vi "niWLAN - OPPO - 80211abgnIQMeasurements.vi"(0 "niwlan analysis session":T5, 2 "Measurement Type":T3(ring), 3 "PL":T2, 7 "TV Parameters(DataType)":T4 {"Standard" items=["80211A/G/J/P OFDM", "80211B/G DSSS", "80211G DSSSOFDM", "80211N MIMOOFDM", "80211AC MIMOOFDM"]; "OFDM Data Rate (Mbps)" items=["6", "9", "12", "18", "24", "36", "48", "54"]; "80211n PLCP Frame Format" items=["Mixed Format", "Greenfield Format"]; "FEC Coding Type" items=["BCC", "LDPC"]; "DSSS Data Rate (Mbps)" items=["1", "2", "5.5 CCK", "5.5 PBCC", "11 CCK", "11 PBCC", "22", "33"]}, 11 "error out":errorcluster) -> (4 "niWLAN session":T5, 6 "Spectrum Result":cluster{"SMM":dbl, "SMM VECTOR":dbl[]}, 8 "Mod Result":T1={"EVM"=-53.23630011850784, "RMS POWER"=-20.854257366141734, "FREQ ERR PPm"=0.0031004693085368165, "Clock ERR PPm"=1.9815491854025864}, 15 "error out":errorcluster)   [LabVIEW 2012]
uses:
  <vilib>/RF Toolkits/WLAN/analysis/controls/wlanv1 Analysis Refnum.ctl
  TV/RW/Includes/WLAN - TV - RW - INC - TV_DataType_Cluster.ctl
  TV/RW/Includes/WLAN - TV - RW - INC - Tx_IQModResult.ctl
  <resource>/objmgr/niWLANAnalysis.rc
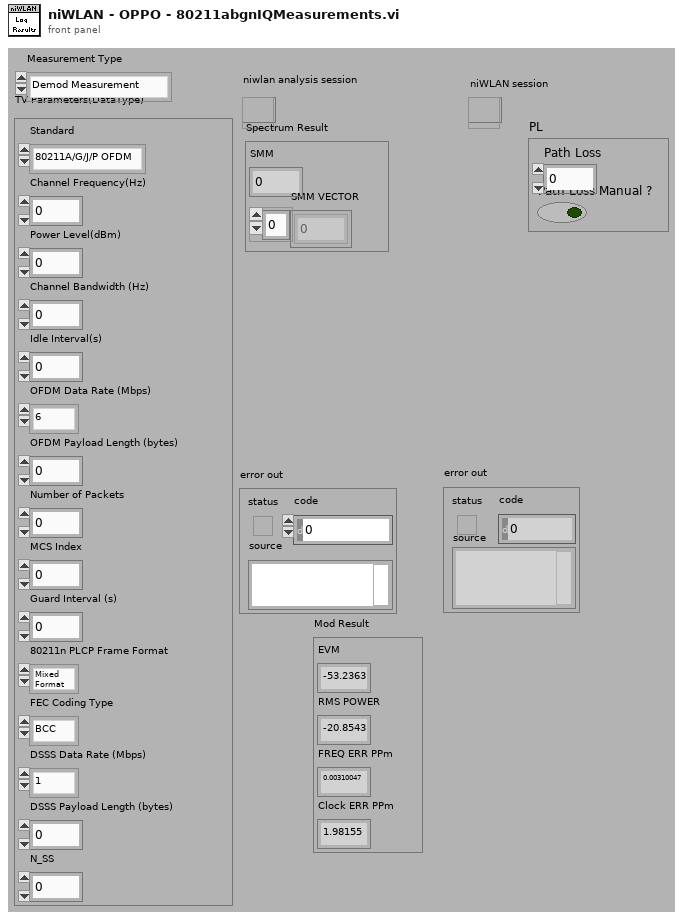
[diagram p1: front panel]
types:
  T1 = typedef "WLAN - TV - RW - INC - Tx_IQModResult.ctl" = cluster{"EVM":dbl, "RMS POWER":dbl, "FREQ ERR PPm":dbl, "Clock ERR PPm":dbl}
  T2 = cluster{"Path Loss":dbl, "Path Loss Manual ?":bool}
  T3 = enum16{"Demod Measurement", "Spectrum Measurement"}
  T4 = typedef "WLAN - TV - RW - INC - TV_DataType_Cluster.ctl" = cluster{"Standard":i32, "Channel Frequency(Hz)":dbl, "Power Level(dBm)":dbl, "Channel Bandwidth (Hz)":dbl, "Idle Interval(s)":dbl, "OFDM Data Rate (Mbps)":i32, "OFDM Payload Length (bytes)":i32, "Number of Packets":i32, "MCS Index":i32, "Guard Interval (s)":dbl, "80211n PLCP Frame Format":i32, "FEC Coding Type":i32, "DSSS Data Rate (Mbps)":i32, "DSSS Payload Length (bytes)":i32, "N_SS":i32}
  T5 = typedef "wlanv1 Analysis Refnum.ctl" = refnum<k20>
  T6 = cluster{"subcarrier indices":i32[], "relative power (dB)":dbl[]}
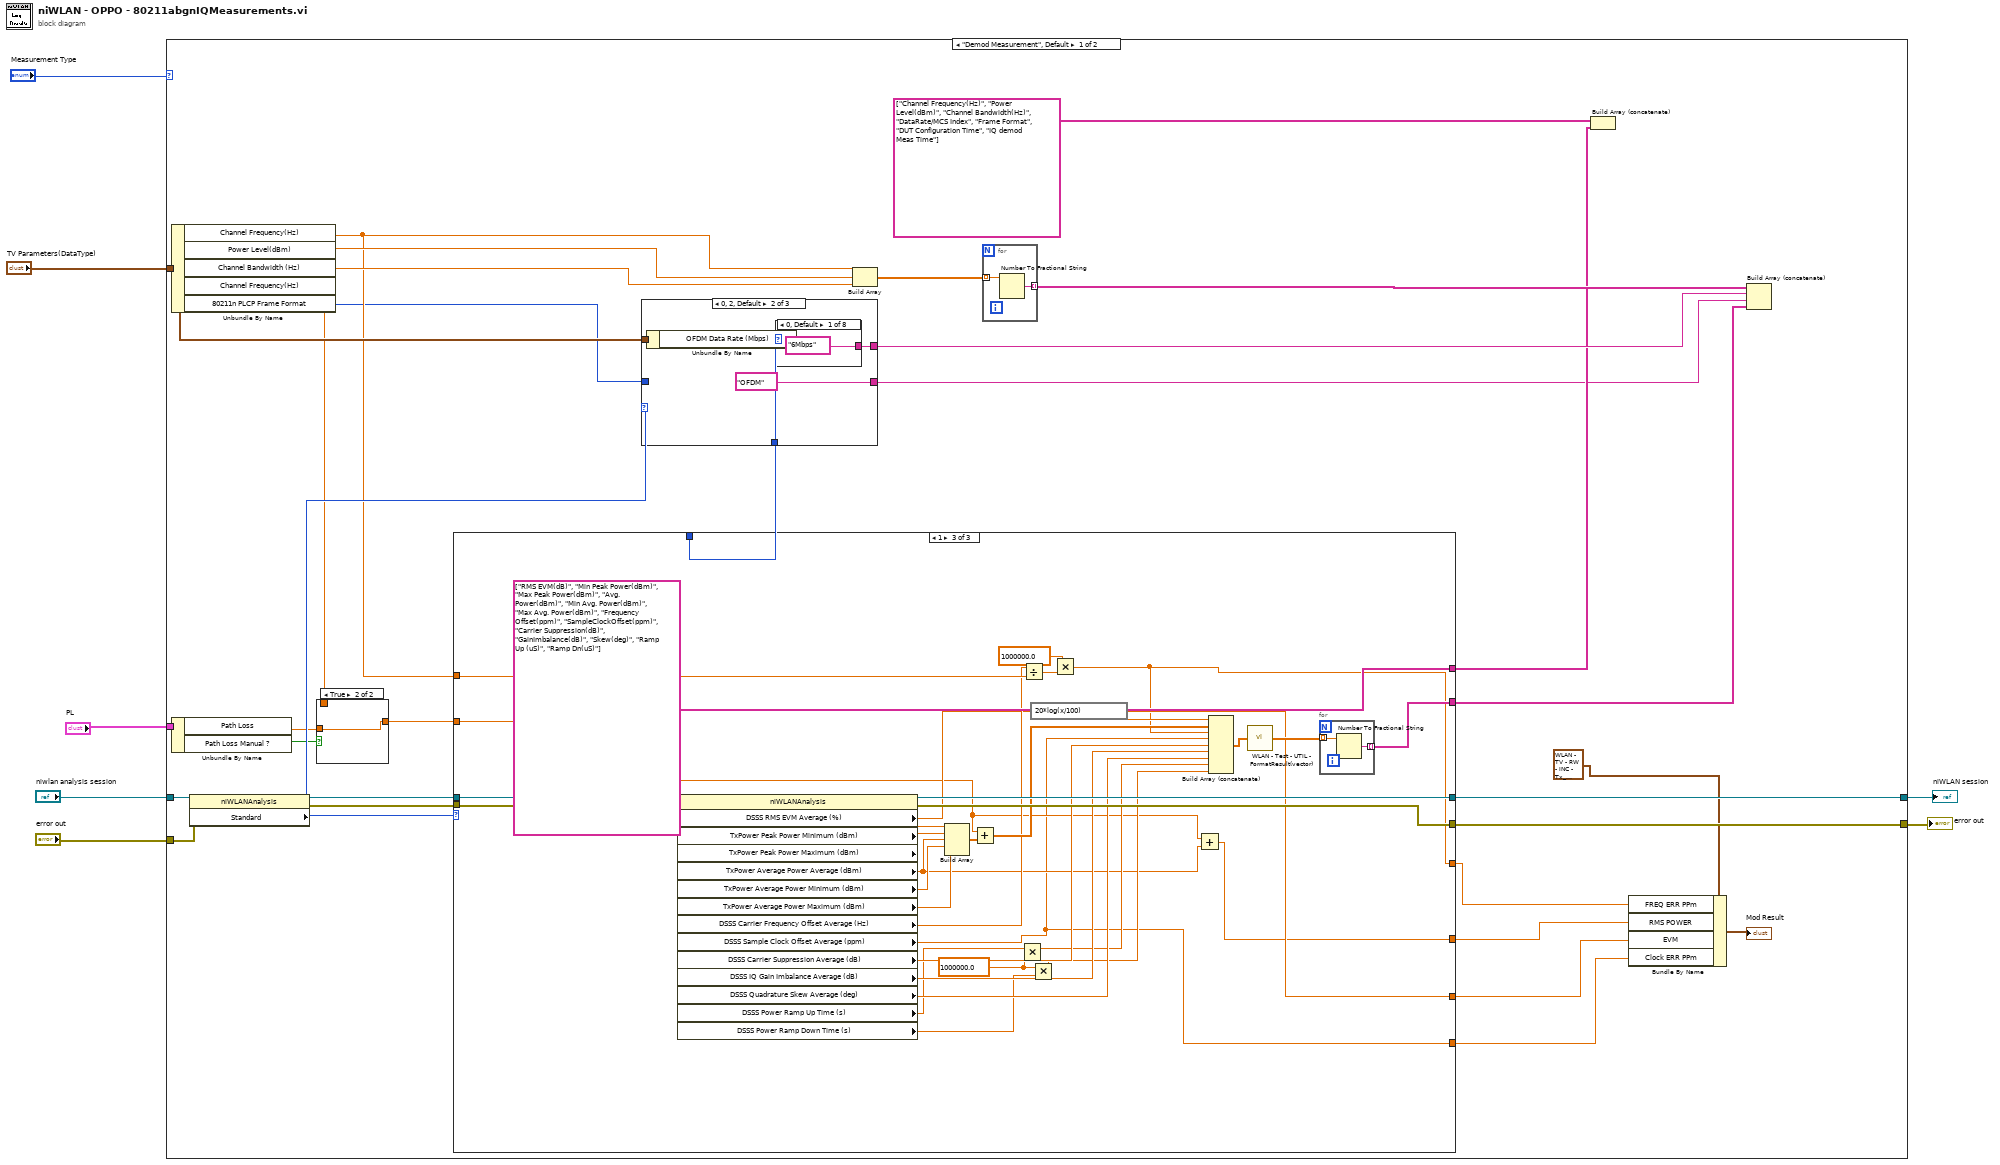
[diagram p0: block diagram]
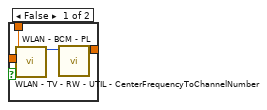
[diagram p2: hidden frame]
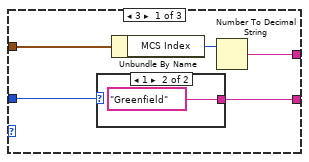
[diagram p3: hidden frame]
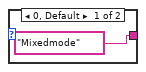
[diagram p4: hidden frame]
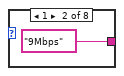
[diagram p5: hidden frame]
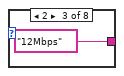
[diagram p6: hidden frame]
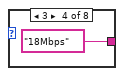
[diagram p7: hidden frame]
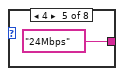
[diagram p8: hidden frame]
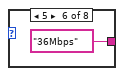
[diagram p9: hidden frame]
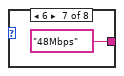
[diagram p10: hidden frame]
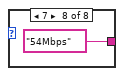
[diagram p11: hidden frame]
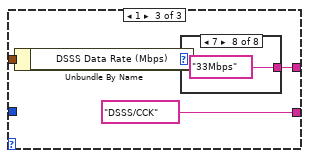
[diagram p12: hidden frame]
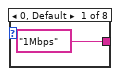
[diagram p13: hidden frame]
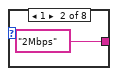
[diagram p14: hidden frame]
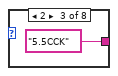
[diagram p15: hidden frame]
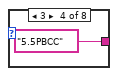
[diagram p16: hidden frame]
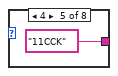
[diagram p17: hidden frame]
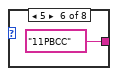
[diagram p18: hidden frame]
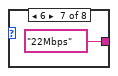
[diagram p19: hidden frame]
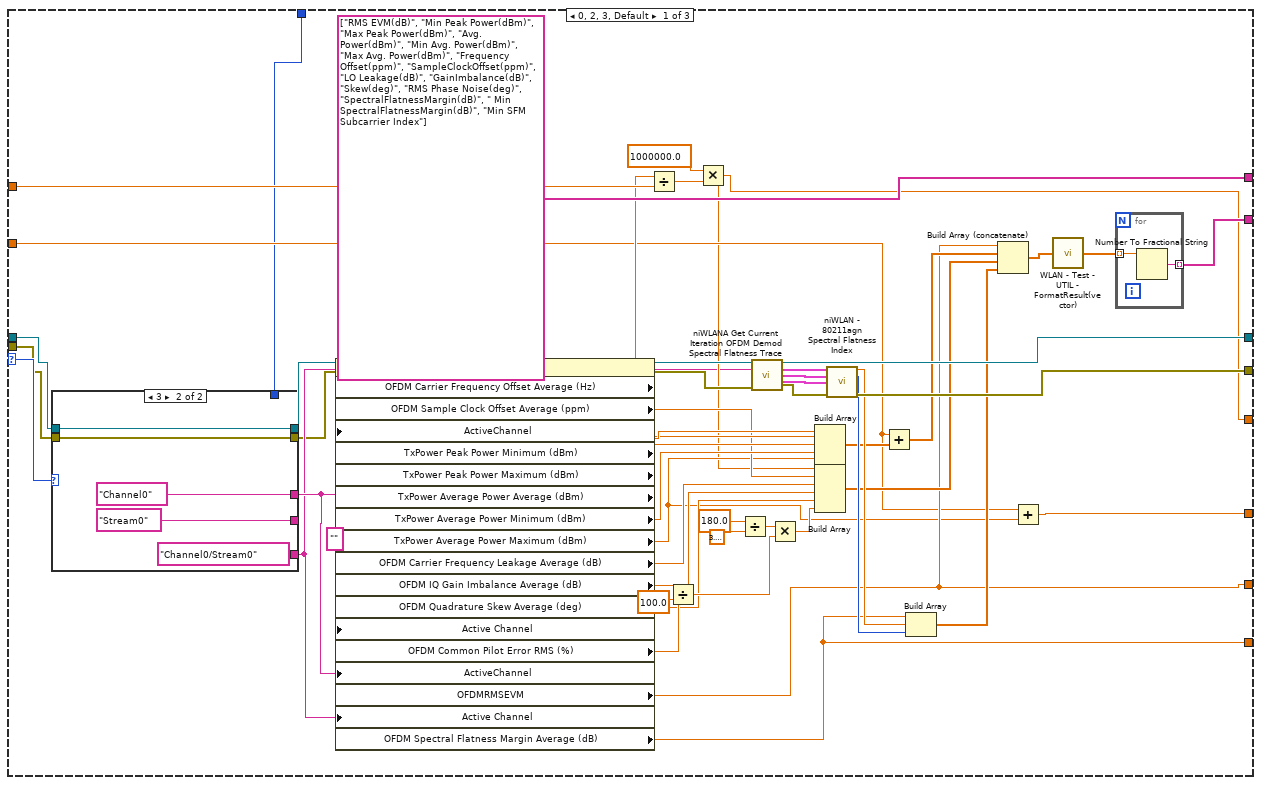
[diagram p20: hidden frame]
diagram:
  n1 = case shown="\"Demod Measurement\", Default" "Measurement Type" {
    tunnel: "niwlan analysis session" -> [w38 w264]
    tunnel: "error out" -> [w36 w265]
    tunnel: "TV Parameters(DataType)" -> [w29 w266]
    tunnel: [w24 w262] -> w4
    tunnel: [w23 w263] -> w3
    tunnel: "PL" -> [w17 _]
    frame "Demod Measurement", Default {
      n2 = Unbundle By Name(w29) -> ("Channel Frequency(Hz)"=w25:dbl, "Power Level(dBm)"=w33:dbl, "Channel Bandwidth (Hz)"=w32:dbl, "Channel Frequency(Hz)"=w20:dbl, "80211n PLCP Frame Format"=w19:i32)
      n3 = Unbundle By Name(w17) -> ("Path Loss"=w15:dbl, "Path Loss Manual ?"=w16:bool)
      n4 = property class="niWLANAnalysis"(reference=w38, error in=w36) -> (reference out=w37:T5, error out=w35:errorcluster, "Standard"=w28:i32)
      n5 = case shown="True" w16 {
        tunnel: [w41 w42] -> w21
        tunnel: w20 -> [w39 _]
        tunnel: w15 -> [_ w42]
        frame False {
          n6 = call "WLAN - TV - RW - UTIL - CenterFrequencyToChannelNumber.vi"("Center Frequency(Hz)"=w39) -> ("Coherced Channel Number"=w40:i32)  [unwired: 13 in, 1 out]
          n7 = call "WLAN - BCM - PL.vi"("Channel index"=w40) -> ("PL"=w41:dbl)  [unwired: 10 in]
        }
        frame True {
        }
      }
      n8 = case shown="1" w28 {
        selector: w28 -> [w127 _ _]
        tunnel: w35 -> [w108 w145 w222]
        tunnel: w37 -> [w77 w146 w223]
        tunnel: [w106 w170 w221] -> w24
        tunnel: [w103 w167 w220] -> w23
        tunnel: [w126 w188 w216] -> w14
        tunnel: [string[] ["RMS EVM(dB)", "Min Peak Power(dBm)", "Max Peak Power(dBm)", "Avg. Power(dBm)", "Min Avg. Power(dBm)", "Max Avg. Power(dBm)", "Frequency Offset(ppm)", "SampleClockOffset(ppm)", "LO Leakage(dB)", "GainImbalance(dB)", "Skew(deg)", "RMS Phase Noise(deg)", "SpectralFlatnessMargin(dB)", " Min SpectralFlatnessMargin(dB)", "Min SFM Subcarrier Index"] string[] ["RMS EVM(dB)", "Min Peak Power(dBm)", "Max Peak Power(dBm)", "Avg. Power(dBm)", "Min Avg. Power(dBm)", "Max Avg. Power(dBm)", "Frequency Offset(ppm)", "SampleClockOffset(ppm)", "LO Leakage(dB)", "GainImbalance(dB)", "Skew(deg)", "RMS Phase Noise(deg)", "SpectralFlatnessMargin(dB)", " Min SpectralFlatnessMargin(dB)", "Min SFM Subcarrier Index"] string[] ["RMS EVM(dB)", "Min Peak Power(dBm)", "Max Peak Power(dBm)", "Avg. Power(dBm)", "Min Avg. Power(dBm)", "Max Avg. Power(dBm)", "Frequency Offset(ppm)", "SampleClockOffset(ppm)", "Carrier Suppression(dB)", "GainImbalance(dB)", "Skew(deg)", "Ramp Up (uS)", "Ramp Dn(uS)"]] -> w26
        tunnel: w25 -> [w122 w184 w215]
        tunnel: [w78 _ _] -> w22
        tunnel: w21 -> [w83 w149 w195]
        tunnel: [w81 w147 w196] -> w12
        tunnel: [w86 w152 w197] -> w10
        tunnel: [w85 w151 w191] -> w13
        tunnel: [w82 w148 w193] -> w11
        frame 0, 2, 3, Default {
          n9 = case shown="3" w127 {
            tunnel: [w135 "Channel0/Stream0"] -> w80
            tunnel: [w135 "Stream0" ("Active Channel")] -> _
            tunnel: [w135 "Channel0" ("Active Channel")] -> w88
            tunnel: w77 -> [w134 w136]
            tunnel: w108 -> [w133 w137]
            tunnel: [w132 w137] -> w79
            tunnel: [w131 _] -> w78
            tunnel: [w130 w136] -> w76
            frame 0, 2, Default {
              w135 = "" ("Active Channel")
              n10 = property class="niWLANAnalysis"(reference=w134, error in=w133) -> (reference out=w130:T5, error out=w132:errorcluster, "Detected OFDM Data Rate (Mbps)"=w131:i32)
            }
            frame 3 {
            }
          }
          n11 = property class="niWLANAnalysis"(reference=w76, error in=w79, "ActiveChannel"=w88, "Active Channel"="", "ActiveChannel"=w88, "Active Channel"=w80) -> (reference out=w107:T5, error out=w105:errorcluster, "OFDM Carrier Frequency Offset Average (Hz)"=w87:dbl, "OFDM Sample Clock Offset Average (ppm)"=w97:dbl, "TxPower Peak Power Minimum (dBm)"=w119:dbl, "TxPower Peak Power Maximum (dBm)"=w118:dbl, "TxPower Average Power Average (dBm)"=w117:dbl, "TxPower Average Power Minimum (dBm)"=w116:dbl, "TxPower Average Power Maximum (dBm)"=w84:dbl, "OFDM Carrier Frequency Leakage Average (dB)"=w96:dbl, "OFDM IQ Gain Imbalance Average (dB)"=w95:dbl, "OFDM Quadrature Skew Average (deg)"=w94:dbl, "OFDM Common Pilot Error RMS (%)"=w109:dbl, "OFDMRMSEVM"=w86:dbl, "OFDM Spectral Flatness Margin Average (dB)"=w85:dbl)
          n12 = Divide(x=w87, y=w122) -> (x/y=w124:dbl)
          n13 = Divide(x=w109, y=100.0 ("x")) -> (x/y=w114:dbl)
          n14 = Multiply(x=1000000.0, y=w124) -> (x*y=w81:dbl)
          n15 = Divide(x=180.0, y=3.141592653589793) -> (x/y=w111:dbl)
          n16 = call <vilib>:"niWLANA Get Current Iteration OFDM Demod Spectral Flatness Trace.vi"("niwlan analysis session"=w107, "active channel"=w80, "error in"=w105) -> ("niwlan analysis session out"=w106:T5, "spectral flatness upper mask"=w102:T6, "spectral flatness trace"=w101:T6, "spectral flatness lower mask"=w100:T6, "error out"=w104:errorcluster)  [unwired: 8 in]
          n17 = Multiply(x=w111, y=w114) -> (x*y=w93:dbl)
          n18 = Build Array(w119, w118, w117, w116, w84) -> (w92:dbl[])
          n19 = Build Array(w81, w97, w96, w95, w94, w93) -> (w89:dbl[])
          n20 = call "niWLAN - 80211agn Spectral Flatness Index.vi"("spectral flatness upper mask"=w102, "spectral flatness Trace"=w101, "spectral flatness Lower mask"=w100, "error in (no error)"=w104) -> ("Least Spectral Flatness Margin"=w98:dbl, "Spectral Flatness Margin Subcarrier Index"=w99:i32, "error out"=w103:errorcluster)  [unwired: 9 in]
          n21 = Add(x=w83, y=w92) -> (x+y=w91:dbl[])
          n22 = Build Array(w85, w98, w99) -> (w90:dbl[])
          n23 = Build Array (concatenate)(w86, w91, w89, w90) -> (w121:dbl[])
          n24 = Add(x=w83, y=w84) -> (x+y=w82:dbl)
          n25 = call "WLAN - Test - UTIL - FormatResult(vector).vi"("Number"=w121) -> ("2nd order decimal"=w120:dbl[])  [unwired: 14 in]
          n26 = for {
            tunnel: [w129] -> w126 mode=indexing
            tunnel: w120 -> [w128] mode=indexing
            n27 = Number To Fractional String(number=w128) -> (F-format string=w129:string)  [unwired: 3 in]
          }
        }
        frame 4 {
          w141 = "Segment0/Channel0/Stream0" ("Active Channel")
          w142 = "Segment0/Channel0" ("Active Channel")
          n28 = property class="niWLANAnalysis"(reference=w146, error in=w145, "Active Channel"="Segment0", "ActiveChannel"=w142, "Active Channel"=w142, "ActiveChannel"=w142, "Active Channel"=w141) -> (reference out=w171:T5, error out=w169:errorcluster, "OFDM Carrier Frequency Offset Average (Hz)"=w144:dbl, "OFDM Sample Clock Offset Average (ppm)"=w161:dbl, "TxPower Peak Power Minimum (dBm)"=w181:dbl, "TxPower Peak Power Maximum (dBm)"=w180:dbl, "TxPower Average Power Average (dBm)"=w179:dbl, "TxPower Average Power Minimum (dBm)"=w178:dbl, "TxPower Average Power Maximum (dBm)"=w150:dbl, "OFDM Carrier Frequency Leakage Average (dB)"=w160:dbl, "OFDM IQ Gain Imbalance Average (dB)"=w159:dbl, "OFDM Quadrature Skew Average (deg)"=w158:dbl, "OFDM Common Pilot Error RMS (%)"=w172:dbl, "OFDMRMSEVM"=w152:dbl, "OFDM Spectral Flatness Margin Average (dB)"=w151:dbl)
          n29 = Divide(x=w144, y=w184) -> (x/y=w186:dbl)
          n30 = Divide(x=w172, y=100.0 ("x")) -> (x/y=w177:dbl)
          n31 = Multiply(x=1000000.0, y=w186) -> (x*y=w147:dbl)
          n32 = Divide(x=180.0, y=3.141592653589793) -> (x/y=w174:dbl)
          n33 = call <vilib>:"niWLANA Get Current Iteration OFDM Demod Spectral Flatness Trace.vi"("niwlan analysis session"=w171, "active channel"=w141, "error in"=w169) -> ("niwlan analysis session out"=w170:T5, "spectral flatness upper mask"=w166:T6, "spectral flatness trace"=w165:T6, "spectral flatness lower mask"=w164:T6, "error out"=w168:errorcluster)  [unwired: 8 in]
          n34 = Multiply(x=w174, y=w177) -> (x*y=w157:dbl)
          n35 = Build Array(w181, w180, w179, w178, w150) -> (w156:dbl[])
          n36 = Build Array(w147, w161, w160, w159, w158, w157) -> (w153:dbl[])
          n37 = call "niWLAN - 80211agn Spectral Flatness Index.vi"("spectral flatness upper mask"=w166, "spectral flatness Trace"=w165, "spectral flatness Lower mask"=w164, "error in (no error)"=w168) -> ("Least Spectral Flatness Margin"=w162:dbl, "Spectral Flatness Margin Subcarrier Index"=w163:i32, "error out"=w167:errorcluster)  [unwired: 9 in]
          n38 = Add(x=w149, y=w156) -> (x+y=w155:dbl[])
          n39 = Build Array(w151, w162, w163) -> (w154:dbl[])
          n40 = Build Array (concatenate)(w152, w155, w153, w154) -> (w183:dbl[])
          n41 = Add(x=w149, y=w150) -> (x+y=w148:dbl)
          n42 = call "WLAN - Test - UTIL - FormatResult(vector).vi"("Number"=w183) -> ("2nd order decimal"=w182:dbl[])  [unwired: 14 in]
          n43 = for {
            tunnel: [w190] -> w188 mode=indexing
            tunnel: w182 -> [w189] mode=indexing
            n44 = Number To Fractional String(number=w189) -> (F-format string=w190:string)  [unwired: 3 in]
          }
        }
        frame 1 {
          w200 = 1000000.0 ("x")
          n45 = property class="niWLANAnalysis"(reference=w223, error in=w222) -> (reference out=w221:T5, error out=w220:errorcluster, "DSSS RMS EVM Average (%)"=w198:dbl, "TxPower Peak Power Minimum (dBm)"=w209:dbl, "TxPower Peak Power Maximum (dBm)"=w208:dbl, "TxPower Average Power Average (dBm)"=w192:dbl, "TxPower Average Power Minimum (dBm)"=w207:dbl, "TxPower Average Power Maximum (dBm)"=w194:dbl, "DSSS Carrier Frequency Offset Average (Hz)"=w199:dbl, "DSSS Sample Clock Offset Average (ppm)"=w191:dbl, "DSSS Carrier Suppression Average (dB)"=w219:dbl, "DSSS IQ Gain Imbalance Average (dB)"=w218:dbl, "DSSS Quadrature Skew Average (deg)"=w217:dbl, "DSSS Power Ramp Up Time (s)"=w204:dbl, "DSSS Power Ramp Down Time (s)"=w203:dbl)
          n46 = Build Array(w209, w208, w192, w207, w194) -> (w206:dbl[])
          n47 = Add(x=w195, y=w206) -> (x+y=w205:dbl[])
          n48 = Multiply(x=w204, y=w200) -> (x*y=w202:dbl)
          n49 = Divide(x=w199, y=w215) -> (x/y=w214:dbl)
          n50 = expression code="20*log(x/100)"(w198) -> (w197:dbl)
          n51 = Multiply(x=w200, y=w203) -> (x*y=w201:dbl)
          n52 = Multiply(x=1000000.0, y=w214) -> (x*y=w196:dbl)
          n53 = Add(x=w195, y=w192) -> (x+y=w193:dbl)
          n54 = Build Array (concatenate)(w197, w205, w196, w191, w219, w218, w217, w202, w201) -> (w211:dbl[])
          n55 = call "WLAN - Test - UTIL - FormatResult(vector).vi"("Number"=w211) -> ("2nd order decimal"=w210:dbl[])  [unwired: 14 in]
          n56 = for {
            tunnel: [w225] -> w216 mode=indexing
            tunnel: w210 -> [w224] mode=indexing
            n57 = Number To Fractional String(number=w224) -> (F-format string=w225:string)  [unwired: 3 in]
          }
        }
      }
      n58 = case shown="0, 2, Default" w28 {
        tunnel: [w47 "OFDM" ("active channel") "DSSS/CCK" ("active channel")] -> w18
        tunnel: w29 -> [w46 w52 w64]
        tunnel: [w44 w51 w62] -> w30
        tunnel: w22 -> [_ w50 _]
        tunnel: w19 -> [w43 _ _]
        frame 3 {
          n59 = case shown="1" w43 {
            tunnel: ["Mixedmode" ("active channel") "Greenfield" ("active channel")] -> w47
            frame 0, Default {
            }
            frame 1 {
            }
          }
          n60 = Unbundle By Name(w46) -> ("MCS Index"=w45:i32)
          n61 = Number To Decimal String(number=w45) -> (decimal integer string=w44:string)  [unwired: 1 in]
        }
        frame 0, 2, Default {
          n62 = Unbundle By Name(w52) -> ()  [unwired: 1 out]
          n63 = case shown="0, Default" w50 {
            tunnel: ["6Mbps" ("active channel") "9Mbps" ("active channel") "12Mbps" ("active channel") "18Mbps" ("active channel") "24Mbps" ("active channel") "36Mbps" ("active channel") "48Mbps" ("active channel") "54Mbps" ("active channel")] -> w51
            frame 0, Default {
            }
            frame 1 {
            }
            frame 2 {
            }
            frame 3 {
            }
            frame 4 {
            }
            frame 5 {
            }
            frame 6 {
            }
            frame 7 {
            }
          }
        }
        frame 1 {
          n64 = Unbundle By Name(w64) -> ("DSSS Data Rate (Mbps)"=w63:i32)
          n65 = case shown="7" w63 {
            tunnel: ["1Mbps" ("active channel") "2Mbps" ("active channel") "5.5CCK" ("active channel") "5.5PBCC" ("active channel") "11CCK" ("active channel") "11PBCC" ("active channel") "22Mbps" ("active channel") "33Mbps" ("active channel")] -> w62
            frame 0, Default {
            }
            frame 1 {
            }
            frame 2 {
            }
            frame 3 {
            }
            frame 4 {
            }
            frame 5 {
            }
            frame 6 {
            }
            frame 7 {
            }
          }
        }
      }
      n66 = Build Array(w25, w33, w32) -> (w34:dbl[])
      n67 = for {
        tunnel: [w75] -> w31 mode=indexing
        tunnel: w34 -> [w74] mode=indexing
        n68 = Number To Fractional String(number=w74) -> (F-format string=w75:string)  [unwired: 3 in]
      }
      n69 = Build Array (concatenate)(string[] ["Channel Frequency(Hz)", "Power Level(dBm)", "Channel Bandwidth(Hz)", "DataRate/MCS Index", "Frame Format", "DUT Configuration Time", "IQ demod Meas Time"], w26) -> ()  [unwired: 1 out]
      n70 = Bundle By Name(cluster=T1 {"EVM"=-53.23630011850784, "RMS POWER"=-20.854257366141734, "FREQ ERR PPm"=0.0031004693085368165, "Clock ERR PPm"=1.9815491854025864} ("Mod Result"), "FREQ ERR PPm"=w12, "RMS POWER"=w11, "EVM"=w10, "Clock ERR PPm"=w13) -> (→"Mod Result":T1)
      n71 = Build Array (concatenate)(w31, w30, w18, w14) -> ()  [unwired: 1 out]
    }
    frame "Spectrum Measurement" {
      n72 = property class="niWLANAnalysis"(reference=w264, error in=w265) -> (reference out=w261:T5, error out=w260:errorcluster, "Standard"=w259:i32)
      n73 = case shown="3" w259 {
        tunnel: ["Channel0" ("active channel") "Segment0/Channel0" ("active channel") "" ("active channel") "" ("active channel")] -> w235
        tunnel: w266 -> [w278 w288 w294 w308]
        tunnel: [w274 w284 w292 w306] -> w237
        tunnel: [string[] ["SMM(-33MHz  -  -30MHz) ", "SMM(dB)(-30MHz  -  -20MHz) ", "SMM(dB)(-20MHz  -  -11MHz) ", "SMM(dB)(-11MHz  -  -9MHz) ", "SMM(dB)(-9MHz  -  9MHz) ", "SMM(dB)(9MHz  -  11MHz) ", "SMM(dB)(11MHz  -  20MHz) ", "SMM(dB)(20MHz  -  30MHz) ", "SMM(dB)(30MHz  -  33MHz) "] string[] ["SMM(-33MHz  -  -30MHz) ", "SMM(dB)(-30MHz  -  -20MHz) ", "SMM(dB)(-20MHz  -  -11MHz) ", "SMM(dB)(-11MHz  -  -9MHz) ", "SMM(dB)(-9MHz  -  9MHz) ", "SMM(dB)(9MHz  -  11MHz) ", "SMM(dB)(11MHz  -  20MHz) ", "SMM(dB)(20MHz  -  30MHz) ", "SMM(dB)(30MHz  -  33MHz) "] string[] ["SMM(-33MHz  -  -30MHz) ", "SMM(dB)(-30MHz  -  -20MHz) ", "SMM(dB)(-20MHz  -  -11MHz) ", "SMM(dB)(-11MHz  -  -9MHz) ", "SMM(dB)(-9MHz  -  9MHz) ", "SMM(dB)(9MHz  -  11MHz) ", "SMM(dB)(11MHz  -  20MHz) ", "SMM(dB)(20MHz  -  30MHz) ", "SMM(dB)(30MHz  -  33MHz) "] string[] ["SMM(-33MHz  -  -22MHz) ", "SMM(-22MHz  -  -11MHz) ", "SMM(-11MHz  -  11MHz) ", "SMM(11MHz  -  22MHz) ", "SMM(22MHz  -  33MHz) "]] -> w234
        tunnel: [w272 "OFDM" ("active channel") "OFDM" ("active channel") "DSSS/CCK" ("active channel")] -> w231
        frame 3 {
          n74 = Unbundle By Name(w278) -> ("MCS Index"=w277:i32, "80211n PLCP Frame Format"=w273:i32)
          n75 = case shown="0, Default" w273 {
            tunnel: ["Mixedmode" ("active channel") "Greenfield" ("active channel")] -> w272
            frame 0, Default {
            }
            frame 1 {
            }
          }
          n76 = Number To Decimal String(number=w277) -> (decimal integer string=w275:string)  [unwired: 1 in]
          n77 = Concatenate Strings("MCS " ("string"), w275) -> (w274:string)
        }
        frame 4 {
          n78 = Unbundle By Name(w288) -> ("MCS Index"=w287:i32)
          n79 = Number To Decimal String(number=w287) -> (decimal integer string=w285:string)  [unwired: 1 in]
          n80 = Concatenate Strings("MCS " ("string"), w285) -> (w284:string)
        }
        frame 0, 2, Default {
          n81 = Unbundle By Name(w294) -> ("OFDM Data Rate (Mbps)"=w293:i32)
          n82 = case shown="7" w293 {
            tunnel: ["6Mbps" ("active channel") "9Mbps" ("active channel") "12Mbps" ("active channel") "18Mbps" ("active channel") "24Mbps" ("active channel") "36Mbps" ("active channel") "48Mbps" ("active channel") "54Mbps" ("active channel")] -> w292
            frame 0, Default {
            }
            frame 1 {
            }
            frame 2 {
            }
            frame 3 {
            }
            frame 4 {
            }
            frame 5 {
            }
            frame 6 {
            }
            frame 7 {
            }
          }
        }
        frame 1 {
          n83 = Unbundle By Name(w308) -> ("DSSS Data Rate (Mbps)"=w307:i32)
          n84 = case shown="7" w307 {
            tunnel: ["1Mbps" ("active channel") "2Mbps" ("active channel") "5.5CCK" ("active channel") "5.5PBCC" ("active channel") "11CCK" ("active channel") "11PBCC" ("active channel") "22Mbps" ("active channel") "33Mbps" ("active channel")] -> w306
            frame 0, Default {
            }
            frame 1 {
            }
            frame 2 {
            }
            frame 3 {
            }
            frame 4 {
            }
            frame 5 {
            }
            frame 6 {
            }
            frame 7 {
            }
          }
        }
      }
      n85 = property class="niWLANAnalysis"(reference=w261, error in=w260, "Active Channel"=w235) -> (reference out=w257:T5, error out=w258:errorcluster, "Spectral Mask Margin (dB)"=w228:dbl, "Spectral Mask Margin Vector"=w227:dbl[])
      n86 = call <vilib>:"niWLANA Get Spectral Mask Trace.vi"("niwlan analysis session"=w257, "active channel"=w235, "error in"=w258) -> ("niwlan analysis session out"=w262:T5, "spectral mask"=w256:cluster{"f0":dbl, "df":dbl, "Y":dbl[]}[], "error out"=w263:errorcluster)  [unwired: 10 in]
      n87 = Index Array(array=w256) -> (element #1=w255:cluster{"f0":dbl, "df":dbl, "Y":dbl[]}, element #2=w254:cluster{"f0":dbl, "df":dbl, "Y":dbl[]})  [unwired: 2 in]
      n88 = Build Array (concatenate)(string[] ["Channel Frequency(Hz)", "Power Level(dBm)", "Channel BW(Hz)", "DataRate/MCS Index", "Frame Format", "DUT Configuration Time", "IQ Spectrum Meas Time", "SM Violation(%) ", "SMM(dB)"], w234) -> ()  [unwired: 1 out]
      n89 = Build Array(w231) -> (w230:string[])
      n90 = Unbundle By Name(w255) -> ("Y"=w253:dbl[])
      n91 = Unbundle By Name(w254) -> ("Y"=w248:dbl[])
      n92 = Subtract(x=w253, y=w248) -> (x-y=w252:dbl[])
      n93 = Array Size(array=w248) -> (size(s)=w247:i32)
      n94 = Less Than 0?(x=w252) -> (x < 0?=w251:bool[])
      n95 = Boolean To (0,1)(Boolean=w251) -> (0, 1=w250:i16[])
      n96 = Add Array Elements(numeric array=w250) -> (sum=w249:i16)
      n97 = Unbundle By Name(w266) -> ("Channel Frequency(Hz)"=w242:dbl, "Power Level(dBm)"=w241:dbl, "Channel Bandwidth (Hz)"=w240:dbl)
      n98 = Divide(x=w249, y=w247) -> (x/y=w246:dbl)
      n99 = Multiply(x=w246, y=100.0) -> (x*y=w244:dbl)
      n100 = Build Array (concatenate)(w244, w228, w227) -> (w233:dbl[])
      n101 = call "WLAN - Test - UTIL - FormatResult(vector).vi"("Number"=w233) -> ("2nd order decimal"=w232:dbl[])  [unwired: 14 in]
      n102 = Build Array(w242, w241, w240) -> (w243:dbl[])
      n103 = for {
        tunnel: [w268] -> w239 mode=indexing
        tunnel: w243 -> [w267] mode=indexing
        n104 = Number To Fractional String(number=w267) -> (F-format string=w268:string)  [unwired: 3 in]
      }
      n105 = for {
        tunnel: [w270] -> w238 mode=indexing
        tunnel: w232 -> [w269] mode=indexing
        n106 = Number To Fractional String(number=w269) -> (F-format string=w270:string)  [unwired: 3 in]
      }
      n107 = Build Array (concatenate)(w239, w237, w230, w238) -> ()  [unwired: 1 out]
      n108 = Bundle By Name(cluster=cluster{"SMM":dbl, "SMM VECTOR":dbl[]} {"SMM"=0.0, "SMM VECTOR"=[]}, "SMM"=w228, "SMM VECTOR"=w227) -> (→"Spectrum Result":cluster{"SMM":dbl, "SMM VECTOR":dbl[]})
    }
  }
  "error out" <- w3
  "niWLAN session" <- w4
